vi "Read Device.vi"(8 "error in (no error)":errorcluster) -> (0 "error out":errorcluster, 2 "Humidity (%RH)":dbl, 3 "Temperature (K)":dbl)   [LabVIEW 2019, in "TEMPerHUM.lvlib"]
uses:
  TEMPerHUM.lvlib
  RDingUSB.dll
panel:
  out "Computer Name":string
  out "Read work?":bool
  out "Write work?":bool
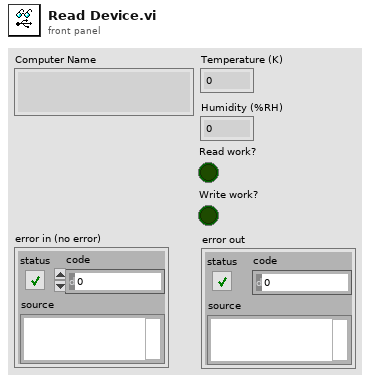
[diagram p1: front panel]
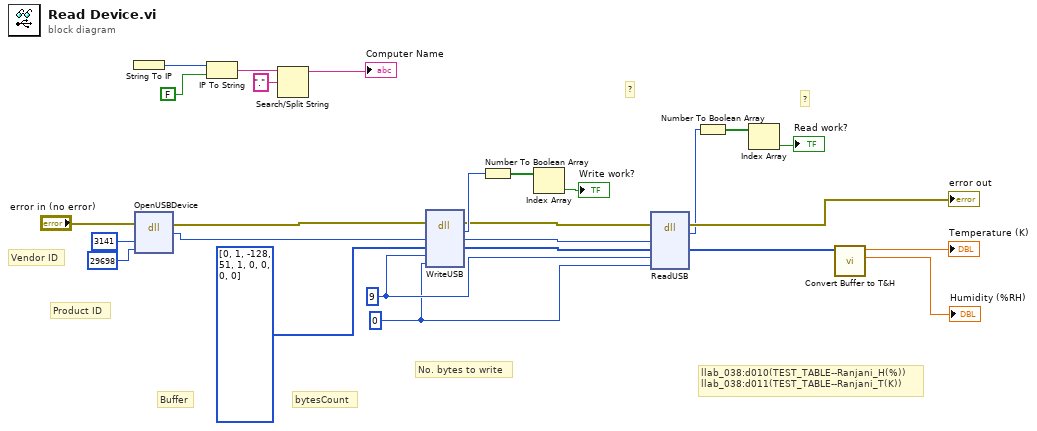
[diagram p0: block diagram]
diagram:
  w11 = u64 0 ("number0fBytesWrite")
  w13 = 9 ("bytesCount")
  # "llab_038:d010(TEST_TABLE--Ranjani_H(%))\nllab_038:d011(TEST_TABLE--Ranjani_T(K))"
  # "bytesCount"
  # "No. bytes to write"
  # "Vendor ID"
  # "Product ID"
  # "Buffer"
  # "?"
  # "?"
  n1 = String To IP() -> (0:w5:u32)  [unwired: 1 in]
  n2 = dll-call lib="C:/Users/Ranjani/Documents/GitHub/Temperhum-Instrument/lvsrc/SMOs/TEMPerHUM/RDingUSB.dll" fn="OpenUSBDevice"(error in="error in (no error)", "VID"=3141, "PID"=29698) -> (error out=w24:errorcluster, "return type"=w25:i64)  [unwired: 4 in, 1 out]
  n3 = IP To String(1:FALSE, 2:w5) -> (0:w3:string)
  n4 = Search/Split String(string=w3, search string/char (-)=".") -> (substring before match=→"Computer Name":string)  [unwired: 1 in, 2 out]
  n5 = dll-call lib="C:/Users/Ranjani/Documents/GitHub/Temperhum-Instrument/lvsrc/SMOs/TEMPerHUM/RDingUSB.dll" fn="WriteUSB"(error in=w24, "deviceHandle"=w25, "buffer"=i8[] [0, 1, -128, 51, 1, 0, 0, 0, 0] ("Array"), "bytesCount"=w13, "number0fBytesWrite"=w11) -> (error out=w9:errorcluster, "return type"=w16:i32, "deviceHandle"=w14:i64, "buffer"=w12:i8[])  [unwired: 4 in, 1 out]
  n6 = Number To Boolean Array(number=w16) -> (Boolean array=w17:bool[])
  n7 = Index Array(array=w17) -> (element=→"Write work?":bool)  [unwired: 1 in]
  n8 = dll-call lib="C:/Users/Ranjani/Documents/GitHub/Temperhum-Instrument/lvsrc/SMOs/TEMPerHUM/RDingUSB.dll" fn="ReadUSB"(error in=w9, "deviceHandle"=w14, "buffer"=w12, "bytesCount"=w13, "number0fBytesRead"=w11) -> (error out=→"error out":errorcluster, "return type"=w21:i32, "buffer"=w22:u8[])  [unwired: 5 in, 1 out]
  n9 = Number To Boolean Array(number=w21) -> (Boolean array=w20:bool[])
  n10 = Index Array(array=w20) -> (element=→"Read work?":bool)  [unwired: 1 in]
  n11 = call "Convert Buffer to T&H.vi"("buffer"=w22) -> ("Humidity"=→"Humidity (%RH)":dbl, "Temperature"=→"Temperature (K)":dbl)  [unwired: 9 in]
